vi "SET_1BIT_Command.vi"(8 "Encender?":bool, 9 "Canal":u8, 10 "Marca":T1) -> (1 "length":i32, 2 "Expected Response":string, 3 "Command":string, 4 "Bytes Expected":u32=2)   [LabVIEW 2019, in "Serial Device.lvclass"]
uses:
  Serial Device.lvclass
  Marca.ctl
  Comando.ctl
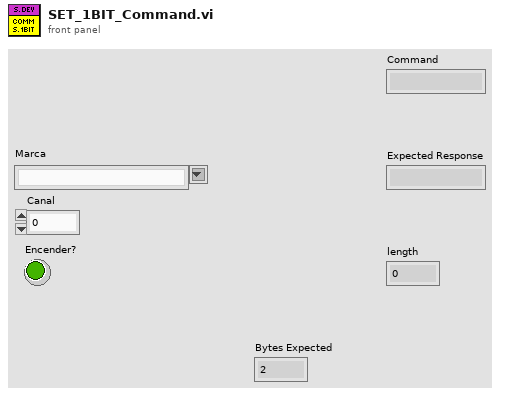
[diagram p1: front panel]
types:
  T1 = typedef "Marca.ctl" = string
  T2 = typedef "Comando.ctl" = string
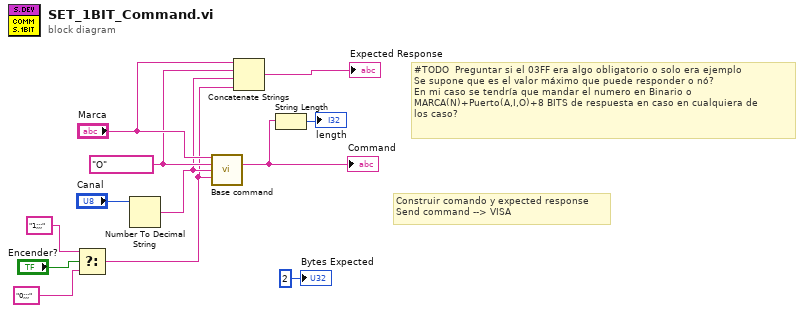
[diagram p0: block diagram]
diagram:
  w10 = T2 "O" ("Comando")
  # "Construir comando y expected response\nSend command --> VISA"
  # "#TODO  Preguntar si el 03FF era algo obligatorio o solo era ejemplo\nSe supone que es el valor máximo que puede responder o nó?\nEn mi caso se tendría que mandar el numero en Binario o \nMARCA(N)+Puerto(A,I,O)+8 BITS de respuesta en caso en cualquiera de \nlos caso?"
  n1 = Select(t="1;;;" ("Parametro 2"), s="Encender?", f="0;;;" ("Parametro 2")) -> (s? t:f=w1:string)
  n2 = Number To Decimal String(number="Canal") -> (decimal integer string=w2:string)  [unwired: 1 in]
  n3 = call "Base command.vi"("Marca"="Marca", "Comando"=w10, "Parametro 1"=w2, "Parametro 2"=w1) -> ("Command"=w8:string)  [unwired: 10 in, 1 out]
  "Command" <- w8
  n4 = Concatenate Strings("Marca", w10, w2, w1) -> (→"Expected Response":string)
  n5 = String Length(string=w8) -> (length=→"length":i32)
  "Bytes Expected" <- u32 2 ("byte count")
